vi "GetFIFOQueue.vi"(4 "ROS":T1={"topic port"=1236, "Node"="/labview", "topic"="/robot/head/command_head_nod", "type"="std_msgs/Bool", "node port"=7000, "error "={"status"=FALSE, "code"=0, "source"=""}, "Direction"=enum."Publisher", "Update (ms)"=1, "FIFO size"=1}) -> (0 "error out":errorcluster, 1 "queue out":refnum<queue>)   [LabVIEW 2018]
doc: "Returns FIFO queue"
uses:
  <userlib>/ROS for LabVIEW Software/ROS/Code/SubVIs/_ROSControl.ctl
  <userlib>/ROS for LabVIEW Software/ROS/Code/SubVIs/_ROSDirection.ctl
  <userlib>/ROS for LabVIEW Software/ROS/Code/_ROSDefinition.vi
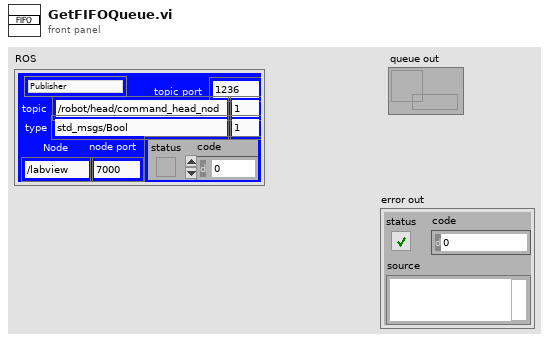
[diagram p1: front panel]
types:
  T1 = typedef "_ROSControl.ctl" = cluster{"topic port":u16, "Node":string, "topic":string, "type":string, "node port":u16, "error ":errorcluster, "Direction":T2, "Update (ms)":u16, "FIFO size":u16}
  T2 = typedef "_ROSDirection.ctl" = enum16{"Node", "Publisher", "Subscriber", "ServiceClient", "ServiceProvider"}
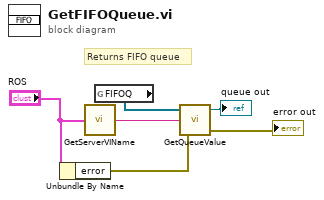
[diagram p0: block diagram]
diagram:
  # "Returns FIFO queue"
  n1 = Unbundle By Name("ROS") -> ("error"=w1:errorcluster)
  n2 = call <userlib>:"GetServerVIName.vi"("ROS"="ROS") -> ("vi name"=w6:string)
  n3 = global read "_ROSDefinition.vi" "FIFOQ"() -> (w2:refnum<queue>[])
  n4 = call <userlib>:"GetQueueValue.vi"("error in"=w1, "vi name"=w6, "Q"=w2) -> ("error out"=→"error out":errorcluster, "Queue out"=→"queue out":refnum<queue>)  [unwired: 1 in]
